vi "Source Voltage_Dual Level.vi"(8 "error in (no error)":errorcluster, 9 "Pins":string[](array[string]), 10 "Voltage Level":dbl[](array[numeric]) format="%_6p", 11 "Semiconductor Module Context":T1) -> (0 "error out":errorcluster, 1 "current measurements":dbl[](array[numeric]), 2 "voltage measurements":dbl[](array[numeric]), 3 "Semiconductor Module Context Out":T1)   [LabVIEW 2013]
uses:
  <vilib>/NI_TestStand_SemiconductorModule/NI_TestStand_Semiconductor_Module.lvlibp/PinMap/General/SemiconductorModuleContext.ctl
  <instrlib>/niDCPower/nidcpower.llb/niDCPower Wait For Event - Event.ctl
  <vilib>/NI_TestStand_SemiconductorModule/NI_TestStand_Semiconductor_Module.lvlibp/PinMap/DC Power/PinsToNIDCPowerSessions.vi
  <vilib>/NI_TestStand_SemiconductorModule/NI_TestStand_Semiconductor_Module.lvlibp
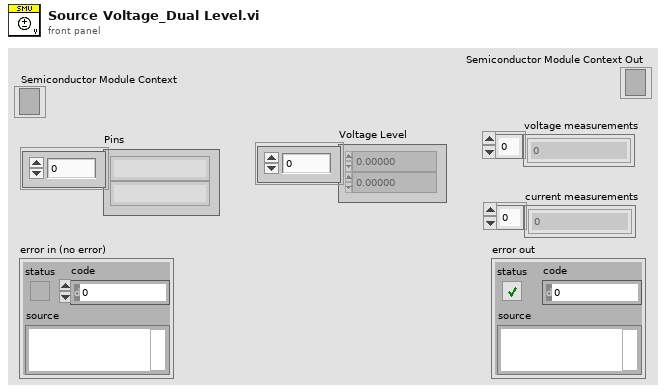
[diagram p1: front panel]
types:
  T1 = typedef "NI_TestStand_Semiconductor_Module.lvlibp/SemiconductorModuleContext.ctl" = refnum<k7>
  T2 = typedef "niDCPower Wait For Event - Event.ctl" = i32
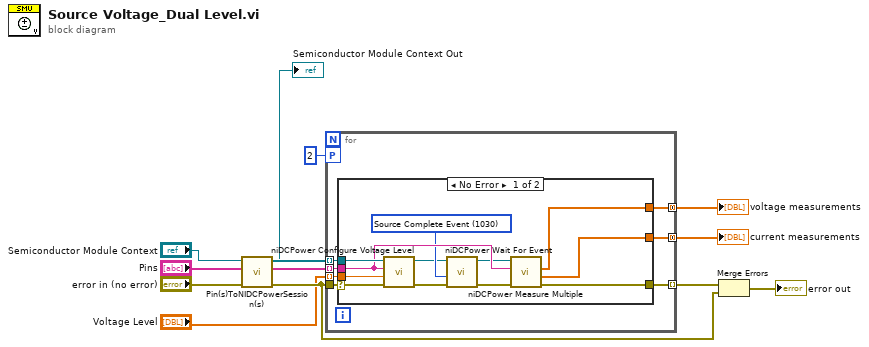
[diagram p0: block diagram]
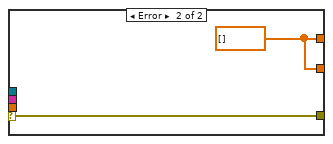
[diagram p2: hidden frame]
diagram:
  n1 = call-poly <vilib>:"Pin(s)ToNIDCPowerSession(s).vi"("error in (no error)"="error in (no error)", "Pins"="Pins", "Semiconductor Module Context"="Semiconductor Module Context") -> ("error out"=w4:errorcluster, "Instrument Sessions"=w12:refnum<k15>[], "Channel Lists"=w11:string[], "Semiconductor Module Context Out"=→"Semiconductor Module Context Out":T1)  [unwired: 4 in, 1 out]
  n2 = for {
    tunnel: "Voltage Level" -> [w20] mode=indexing
    tunnel: w12 -> [w19] mode=indexing
    tunnel: w11 -> [w18] mode=indexing
    tunnel: [w17] -> w9 mode=concatenating
    tunnel: w4 -> [w16]
    tunnel: [w15] -> w8 mode=concatenating
    tunnel: [w14] -> w6 mode=indexing
    workers-P: 2 -> [_]
    n3 = case shown="No Error" w16 {
      selector: w16 -> [w29 w34]
      tunnel: [w21 w34] -> w14
      tunnel: w19 -> [w32 _]
      tunnel: w18 -> [w31 _]
      tunnel: w20 -> [w30 _]
      tunnel: [w23 w33] -> w15
      tunnel: [w22 w33] -> w17
      frame No Error {
        w27 = T2 1030 items=["Source Complete Event"=1030, "Measure Complete Event"=1031, "Sequence Iteration Complete Event"=1032, "Sequence Engine Done Event"=1033, "Pulse Complete Event"=1051, "Ready For Pulse Trigger Event"=1052] ("event")
        n4 = call <instrlib>:"niDCPower Configure Voltage Level.vi"("error in (no error)"=w29, "voltage level"=w30, "channel name"=w31, "instrument handle"=w32) -> ("error out"=w28:errorcluster, "instrument handle out"=w26:refnum<k15>)  [unwired: 6 in]
        n5 = call <instrlib>:"niDCPower Wait For Event.vi"("error in (no error)"=w28, "event"=w27, "instrument handle"=w26) -> ("error out"=w25:errorcluster, "instrument handle out"=w24:refnum<k15>)  [unwired: 7 in]
        n6 = call <instrlib>:"niDCPower Measure Multiple.vi"("error in (no error)"=w25, "channel name"=w31, "instrument handle"=w24) -> ("error out"=w21:errorcluster, "current measurements"=w22:dbl[], "voltage measurements"=w23:dbl[])  [unwired: 5 in, 1 out]
      }
      frame Error {
        w33 = dbl[] [] ("voltage measurements")
      }
    }
  }
  "voltage measurements" <- w8
  "current measurements" <- w9
  n7 = Merge Errors(w6, w4) -> (→"error out":errorcluster)
